vi "testPython.vi"(11 "Path to script":path) -> ()   [LabVIEW 2016]
panel:
  in  "command line":string
  out "command line output":string
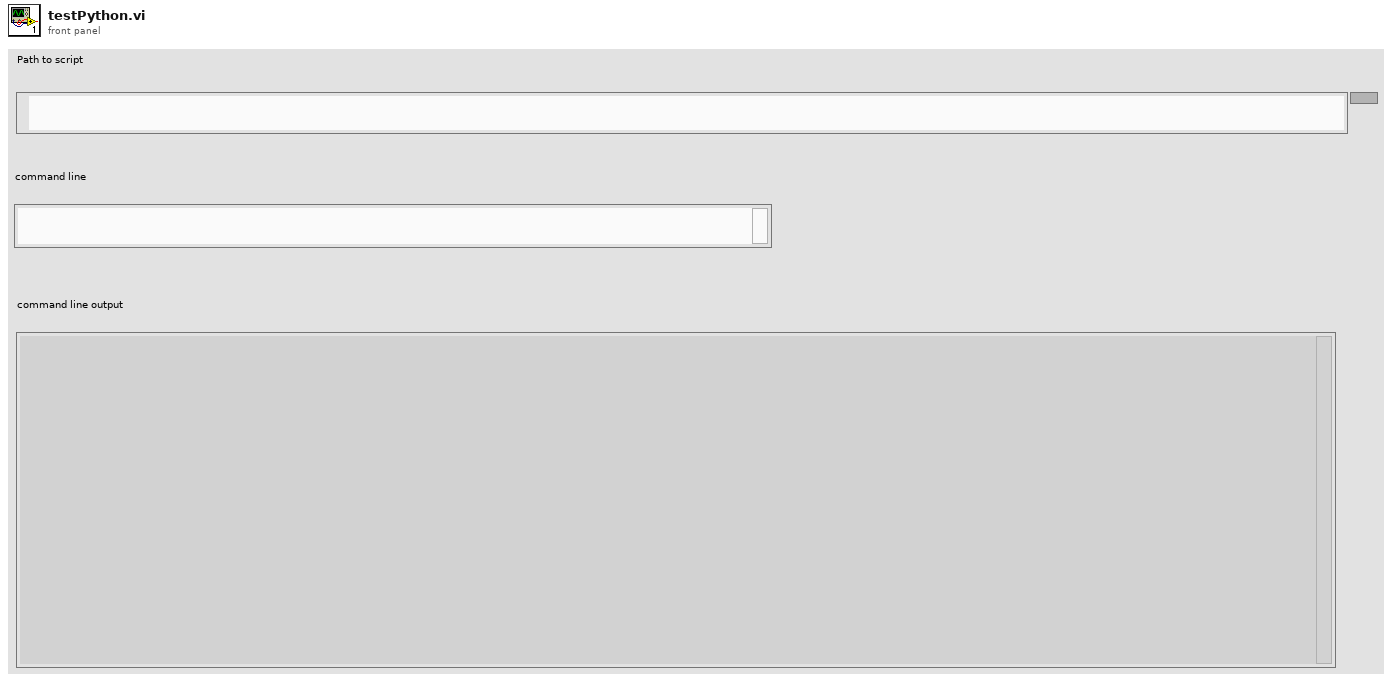
[diagram p1: front panel]
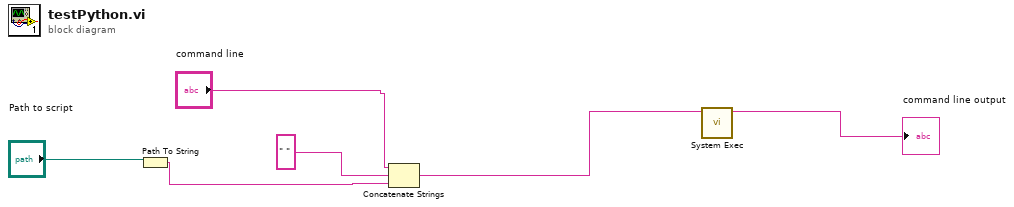
[diagram p0: block diagram]
diagram:
  n1 = Path To String(path="Path to script") -> (string=w5:string)
  n2 = Concatenate Strings("command line", " " ("string"), w5) -> (w2:string)
  n3 = call <vilib>:"System Exec.vi"("command line"=w2) -> ("standard output"=→"command line output":string)  [unwired: 7 in, 3 out]
